vi "Periodic Tasks.vi"(8 "error in":errorcluster) -> ()   [LabVIEW 2019]
doc: "This VI runs in parallel to other tasks. It can contain as many user-defined periodic loops as you need. These can carry out PID or other sorts of timed response."
uses:
  gyro sensor NavX/_TypeDefs/FRIC_navX_DeviceNumbersTypeDef.ctl
  Functions/Global Variables/Trajectory Enabled.vi
  <vilib>/Rock Robotics/Network Tables/NT Write Boolean.vi
  Functions/Global Variables/reset gyro.vi
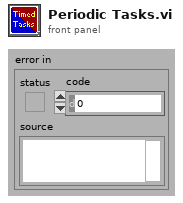
[diagram p1: front panel]
types:
  T1 = typedef "WPI_JoystickDevRef.ctl" = cluster{"Device":T2}
  T2 = typedef "WPI_JoystickDeviceEnum.ctl" = enum16{"USB 0", "USB 1", "USB 2", "USB 3", "USB 4", "USB 5"}
  T3 = typedef "Robot Actions Array.ctl" = T4[]
  T4 = typedef "Robot Actions.ctl" = cluster{"Durations":dbl, "Robot State":T5, "DriveJoystickButtonMapping":T13}
  T5 = typedef "Robot State.ctl" = cluster{"Drive System State":T6, "Enable Actions":T9, "Lift System Actions":T10, "SpinnerActions":T11, "Ball System Actions":T12, "Camera Control":bool}
  T6 = typedef "Robot Pivot Motion Commands.ctl" = cluster{"Front Right":T7, "Front Left":T7, "Rear Left":T7, "Rear Right":T7, "Drive Mode":T8, "Reset Drive Encoder":bool}
  T7 = typedef "Pivot Motor Commands.ctl" = cluster{"Drive Power":dbl, "Drive Distance (in)":dbl, "Drive Distance Error (in)":dbl, "Steer Power":dbl, "Steer Angle (deg)":dbl, "Steer Angle Error (deg)":dbl}
  T8 = typedef "Robot Drive Mode.ctl" = enum16{"Velocity", "Distance"}
  T9 = typedef "Enable Actions.ctl" = cluster{"Manual Swerve Drive":bool, "Color System":bool, "Ball System":bool, "Lift System":bool}
  T10 = typedef "Lift System Actions.ctl" = cluster{"Arm Deploy Piston":bool, "Enable Lift Arm":bool, "Enable Climber":bool, "Climber Velocity":dbl, "Lift Arm Velocity":dbl}
  T11 = typedef "Spinner Actions.ctl" = cluster{"Manual Mode ":bool, "Auto rotate n times":bool, "Auto rotate to color\t":bool, "Extend and Retract Arm\t":bool, "Manual Rotation Speed":dbl}
  T12 = typedef "Ball System Actions.ctl" = cluster{"Intake Piston ":bool, "Shoot Ball":bool, "Tube up one Increment\t":bool, "Reverse Ball Intake":bool, "Tube Piston":bool, "Enable Manual Tube":bool, "Tube up four Increments":bool, "Manual Tube Velocity":dbl, "Ball Intake Speed":dbl, "Color Wheel (Shooter)":bool, "Reverse Shooter":bool}
  T13 = typedef "DriveJoystickData.ctl" = cluster{"Relative Encoders?":bool, "Zero Steer Encoder":bool, "Reset Field Orientation":bool, "Use Field Orientation":bool, "Drive X":dbl, "Drive Y":dbl, "Drive Z":dbl, "Fast Speed Accelerator":dbl, "Increase Max Speed":bool, "Decrease Max Speed":bool, "Camera Controller":bool, "Intake Speed":dbl, "Tube Piston":bool}
  T14 = typedef "FRIC_navX_DeviceNumbersTypeDef.ctl" = enum16{"Dev0", "Dev1", "Dev2", "Dev3"}
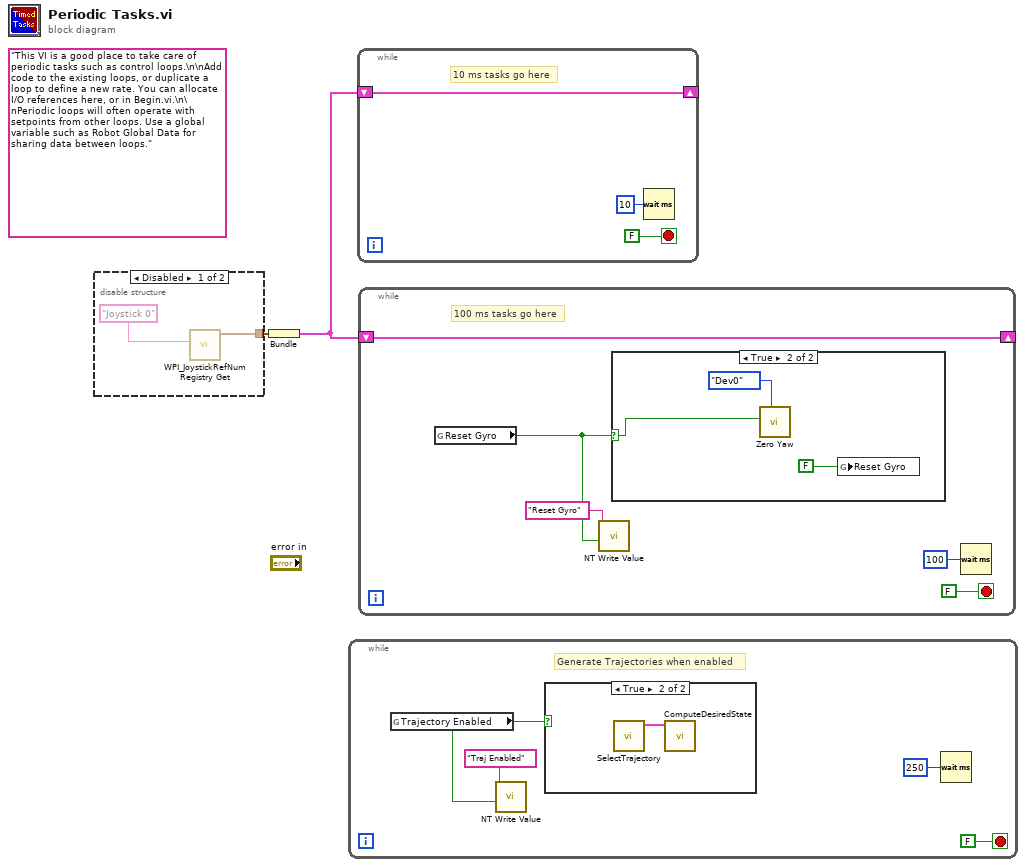
[diagram p0: block diagram]
diagram:
  (unwired) "This VI is a good place to take care of periodic tasks such as control loops.\n\nAdd code to the existing loops, or duplicate a loop to define a new rate. You can allocate I/O references here, or in Begin.vi.\n\nPeriodic loops will often operate with setpoints from other loops. Use a global variable such as Robot Global Data for sharing data between loops."
  n1 = disable-structure shown="Disabled" {
    disable-tunnel: [w3 _] -> w2
    frame Disabled {
      n2 = call <vilib>:"WPI_JoystickRefNum Registry Get.vi"("refnum name"="Joystick 0") -> ("JoystickDevRef"=w3:T1)  [unwired: 1 in, 9 out]
    }
    frame Enabled {
    }
  }
  n3 = Bundle("JoystickDevRef"=w2) -> (w1:cluster{"JoystickDevRef":T1})  [unwired: 1 out]
  n4 = while {
    stop <- FALSE stop-if-true
    # "Generate Trajectories when enabled"
    n5 = global read "Trajectory Enabled.vi" "Trajectory Enabled"() -> (w5:bool)
    n6 = call-poly <vilib>:"NT Write Value.vi"("Boolean"=w5, "Name"="Traj Enabled") -> ()  [unwired: 9 in, 1 out]
    n7 = case shown="True" w5 {
      frame False {
      }
      frame True {
        n8 = call "SelectTrajectory.vi"() -> ("Robot Action Array"=w9:T3)  [unwired: 11 in]
        n9 = call "ComputeDesiredState.vi"("Robot Action Array"=w9) -> ()  [unwired: 11 in]
      }
    }
    n10 = Wait (ms)(milliseconds to wait=u32 250) -> ()  [unwired: 1 out]
  }
  n11 = while {
    shift-right: [w10] -> _
    shift-left: w1 -> [w10]
    stop <- FALSE stop-if-true
    # "10 ms tasks go here"
    n12 = Wait (ms)(milliseconds to wait=u32 10) -> ()  [unwired: 1 out]
  }
  n13 = while {
    shift-right: [w15] -> _
    shift-left: w1 -> [w15]
    stop <- FALSE stop-if-true
    # "100 ms tasks go here"
    n14 = global read "reset gyro.vi" "Reset Gyro"() -> (w14:bool)
    n15 = call-poly <vilib>:"NT Write Value.vi"("Boolean"=w14, "Name"="Reset Gyro") -> ()  [unwired: 9 in, 1 out]
    n16 = case shown="True" w14 {
      selector: w14 -> [_ w19]
      frame False {
      }
      frame True {
        n17 = call "Zero Yaw.vi"("Device Number"=FRIC_navX_DeviceNumbersTypeDef."Dev0", "Zero"=w19) -> ()  [unwired: 10 in]
        n18 = global write "reset gyro.vi" "Reset Gyro"(FALSE ("Reset Gyro")) -> ()
      }
    }
    n19 = Wait (ms)(milliseconds to wait=u32 100) -> ()  [unwired: 1 out]
  }
